vi "Agilent SNA Read Sweep Type.vi"(6 "Channel":i8=1 min=1 max=99 step=1, 7 "Agilent SNA & SWP":T1, 8 "error in (no error)":errorcluster, 11 "VISA Resource Names":T2) -> (0 "error out":errorcluster, 2 "Sweep Type":T3, 3 "dup VISA Resource Names":T2)   [LabVIEW 2011]
doc: "This VI for the HP 8753 is used to read the sweep type.\n\n0 LINEAR FREQ\n1 LOG FREQ\n2 LIST FREQ\n3 CW TIME\n4 POWER SWEEP"
uses:
  TypeDefs/Agilent SNA Sweep Type.ctl
  TypeDefs/Agilent SNA VISA.ctl
  TypeDefs/Agilent SNA Instrument Info.ctl
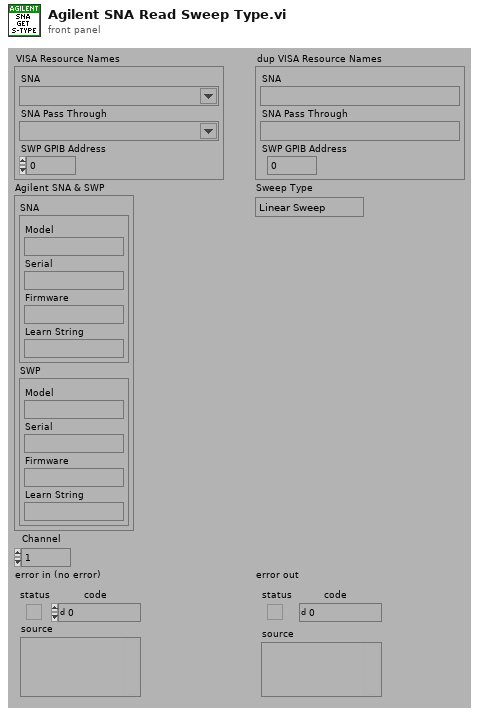
[diagram p1: front panel]
types:
  T1 = typedef "Agilent SNA Instrument Info.ctl" = cluster{"SNA":cluster{"Model":string, "Serial":string, "Firmware":string, "Learn String":string}, "SWP":cluster{"Model":string, "Serial":string, "Firmware":string, "Learn String":string}}
  T2 = typedef "Agilent SNA VISA.ctl" = cluster{"SNA":refnum<visa-resource-name>, "SNA Pass Through":refnum<visa-resource-name>, "SWP GPIB Address":i32}
  T3 = typedef "Agilent SNA Sweep Type.ctl" = enum32{"Linear Sweep", "CW Time Sweep", "Frequency List"}
  T4 = typedef "Agilent SNA Model.ctl" = enum16{"Not Supported", "8757X"}
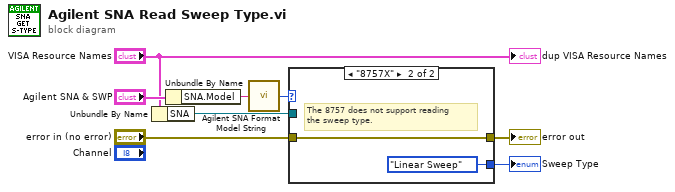
[diagram p0: block diagram]
diagram:
  n1 = Unbundle By Name("VISA Resource Names") -> ("SNA"=w1:refnum<visa-resource-name>)
  n2 = Unbundle By Name("Agilent SNA & SWP") -> ("SNA.Model"=w3:string)
  n3 = call "Agilent SNA Format Model String.vi"("Model String"=w3) -> ("Model"=w5:T4)
  n4 = case shown="\"8757X\"" w5 {
    tunnel: "error in (no error)" -> [w9 w10]
    tunnel: [w9 w10] -> w7
    tunnel: [_ Agilent_SNA_Sweep_Type."Linear Sweep" ("sweep type")] -> w6
    tunnel: w1 -> [_ _]
    frame "Not Supported" {
    }
    frame "8757X" {
      # "The 8757 does not support reading\nthe sweep type."
    }
  }
  "Sweep Type" <- w6
  "error out" <- w7
  "dup VISA Resource Names" <- "VISA Resource Names"
